vi "Get Step Prompt.vi"(0 "VISA resource name":refnum<visa-resource-name>, 11 "error in (no error)":errorcluster) -> (4 "VISA resource name out":refnum<visa-resource-name>, 6 "Prompt":string, 15 "error out":errorcluster)   [LabVIEW 2016, in "APT 300XAC Series.lvlib"]
doc: "Gets the Step Prompt set to the active step of the Power source instrument.\n\nNiote : Only for Program mode. Make sure the instrument is set to the program mode and then the prefered step for prompt is set as the active step."
uses:
  APT 300XAC Series.lvlib
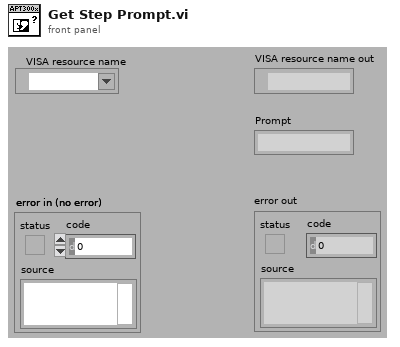
[diagram p1: front panel]
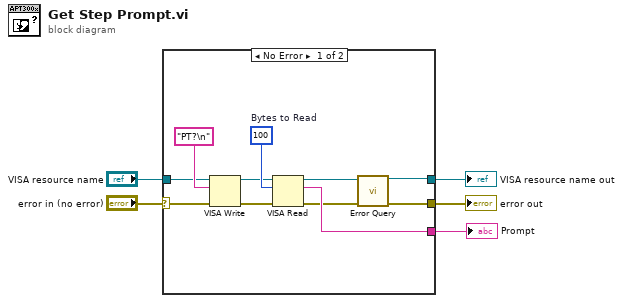
[diagram p0: block diagram]
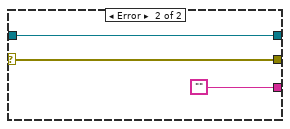
[diagram p2: hidden frame]
diagram:
  n1 = case shown="No Error" "error in (no error)" {
    selector: "error in (no error)" -> [w12 w19]
    tunnel: [w9 w19] -> w4
    tunnel: [w8 w18] -> w2
    tunnel: "VISA resource name" -> [w11 w18]
    tunnel: [w10 ""] -> w1
    frame No Error {
      w16 = u32 100  # Bytes to Read
      n2 = VISA Write(VISA resource name=w11, write buffer="PT?\n", error in (no error)=w12) -> (VISA resource name out=w14:refnum<visa-resource-name>, error out=w15:errorcluster)  [unwired: 1 out]
      n3 = VISA Read(VISA resource name=w14, byte count=w16, error in (no error)=w15) -> (VISA resource name out=w7:refnum<visa-resource-name>, read buffer=w10:string, error out=w6:errorcluster)  [unwired: 1 out]
      n4 = call "Error Query.vi"("VISA resource name"=w7, "error in (no error)"=w6) -> ("VISA resource name out"=w8:refnum<visa-resource-name>, "error out"=w9:errorcluster)  [unwired: 10 in, 2 out]
    }
    frame Error {
    }
  }
  "error out" <- w4
  "VISA resource name out" <- w2
  "Prompt" <- w1
